vi "deadband.vi"() -> ()   [LabVIEW 2010, in "Demobot.lvrbt"]
uses:
  Demobot.lvrbt
panel:
  out "A 2":i32
  out "B 2":i32
  in  "Deadband":dbl
  in  "B":i32
  in  "C":i32
  in  "D":i32
  in  "A":i32
  out "C2":i32
  out "D2":i32
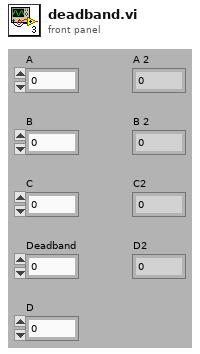
[diagram p1: front panel]
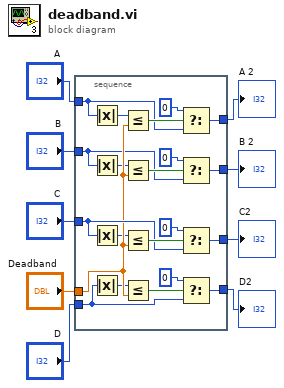
[diagram p0: block diagram]
diagram:
  n1 = stacked-sequence {
    tunnel: "A" -> [w10]
    tunnel: "B" -> [w11]
    tunnel: "C" -> [w22]
    tunnel: "D" -> [w21]
    tunnel: [w20] -> w2
    tunnel: [w19] -> w1
    tunnel: [w18] -> w8
    tunnel: [w17] -> w9
    tunnel: "Deadband" -> [w16]
    frame #0 {
      n2 = Absolute Value(x=w10) -> (abs(x)=w14:i32)
      n3 = Absolute Value(x=w11) -> (abs(x)=w15:i32)
      n4 = Absolute Value(x=w22) -> (abs(x)=w13:i32)
      n5 = Absolute Value(x=w21) -> (abs(x)=w12:i32)
      n6 = Less Or Equal?(x=w14, y=w16) -> (x <= y?=w30:bool)
      n7 = Less Or Equal?(x=w15, y=w16) -> (x <= y?=w27:bool)
      n8 = Less Or Equal?(x=w13, y=w16) -> (x <= y?=w25:bool)
      n9 = Less Or Equal?(x=w12, y=w16) -> (x <= y?=w24:bool)
      n10 = Select(t=0, s=w30, f=w10) -> (s? t:f=w19:i32)
      n11 = Select(t=0, s=w27, f=w11) -> (s? t:f=w20:i32)
      n12 = Select(t=0, s=w25, f=w22) -> (s? t:f=w18:i32)
      n13 = Select(t=0, s=w24, f=w21) -> (s? t:f=w17:i32)
    }
  }
  "D2" <- w9
  "C2" <- w8
  "B 2" <- w2
  "A 2" <- w1
